vi "Write Variable.vi"   [LabVIEW 2016, in "LV-Data.PGSQL.lvclass"]
uses:
  LV-Data.PGSQL.lvclass
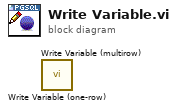
[diagram p0: block diagram]
diagram:
  n1 = call "Write Variable (one-row).vi"() -> ()  [unwired: 9 in, 3 out]
  n2 = call "Write Variable (multirow).vi"() -> ()  [unwired: 9 in, 3 out]
